vi "Read Synchronous Display.vi"(8 "error in (no error)":errorcluster, 11 "Control.lvclass in":refnum<class "Control.lvclass">) -> (0 "error out":errorcluster, 2 "SyncDisp":bool, 3 "Control.lvclass out":refnum<class "Control.lvclass">)   [LabVIEW 2015, in "Control.lvclass"]
uses:
  Control.lvclass
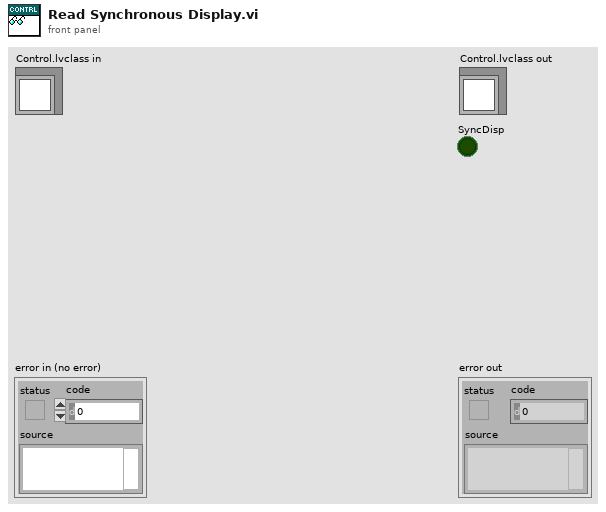
[diagram p1: front panel]
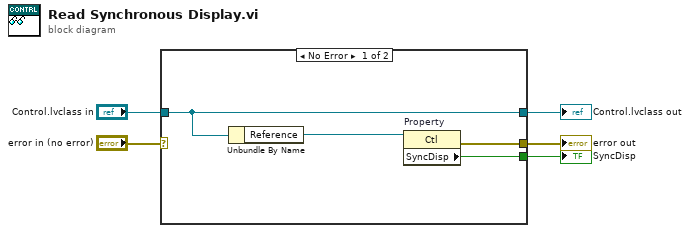
[diagram p0: block diagram]
diagram:
  n1 = case shown="No Error" "error in (no error)" {
    selector: "error in (no error)" -> [_ w11]
    tunnel: [w8 w11] -> w4
    tunnel: [w7 w10] -> w2
    tunnel: "Control.lvclass in" -> [w7 w10]
    tunnel: [w9 _] -> w1
    frame No Error {
      n2 = Unbundle By Name(w7) -> ("Reference"=w6:refnum<vi>)
      n3 = property on="Property" class="Ctl"(reference=w6) -> (error out=w8:errorcluster, "SyncDisp"=w9:bool)  [unwired: 1 in, 1 out]
    }
    frame Error {
    }
  }
  "error out" <- w4
  "Control.lvclass out" <- w2
  "SyncDisp" <- w1
